vi "Pre Launch Init.vi"(11 "UI in":refnum<class "UI.lvclass">) -> (0 "error out":errorcluster, 3 "UI out":refnum<class "UI.lvclass">)   [LabVIEW 2020, in "UI.lvlib" / "UI.lvclass"]
doc: "<p>(<strong>Filename</strong>: <span class=\"dnl\">Actor Framework.lvlib:Actor.lvclass:Pre Launch Init.vi</span>)</p>\n<p>Defines behavior that occurs after the <a href=\"nihelplauncher://docs/csh?context=lvcore_lvcomm_af_launch_nested_actor\">Launch Nested Actor</a> method is invoked but before the actor's Actor Core method begins running.</p>\n<p>By default, this method does nothing. A descendant class may override it to define behavior.</p>"
uses:
  UI.lvclass
  UI.lvclass/UI.ctl
  <vilib>/ActorFramework/Actor/Actor.lvclass
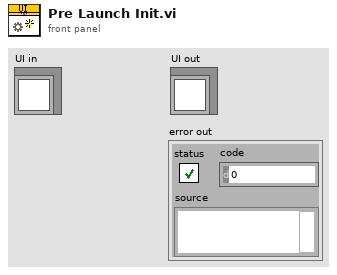
[diagram p1: front panel]
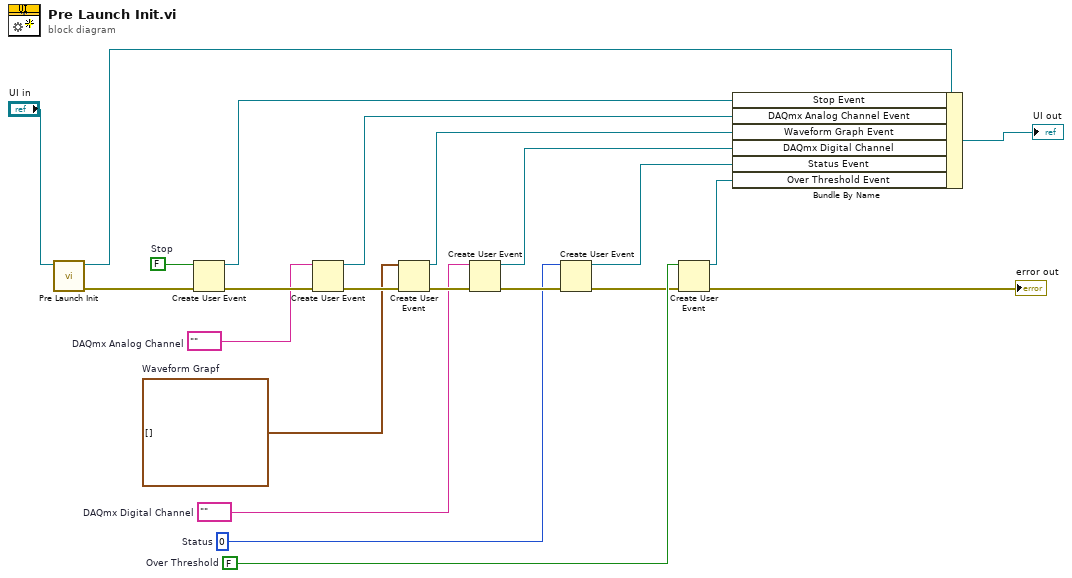
[diagram p0: block diagram]
diagram:
  w4 = FALSE  # Over Threshold
  w6 = waveform(dbl)[] []  # Waveform Grapf
  w8 = u8 0  # Status
  w10 = tag ""  # DAQmx Digital Channel
  w12 = tag ""  # DAQmx Analog Channel
  w14 = FALSE  # Stop
  n1 = call-parent "Pre Launch Init.vi"("Actor in"="UI in") -> ("error out"=w15:errorcluster, "Actor out"=w21:refnum<class "UI.lvclass">)  [unwired: 9 in]
  n2 = Create User Event(user event datatype=w14, error in=w15) -> (user event=w13:refnum<user-event>, error out=w19:errorcluster)
  n3 = Create User Event(user event datatype=w12, error in=w19) -> (user event=w11:refnum<user-event>, error out=w18:errorcluster)
  n4 = Create User Event(user event datatype=w6, error in=w18) -> (user event=w5:refnum<user-event>, error out=w17:errorcluster)
  n5 = Create User Event(user event datatype=w10, error in=w17) -> (user event=w9:refnum<user-event>, error out=w16:errorcluster)
  n6 = Create User Event(user event datatype=w8, error in=w16) -> (user event=w7:refnum<user-event>, error out=w3:errorcluster)
  n7 = Create User Event(user event datatype=w4, error in=w3) -> (user event=w2:refnum<user-event>, error out=→"error out":errorcluster)
  n8 = Bundle By Name(cluster=w21, "Stop Event"=w13, "DAQmx Analog Channel Event"=w11, "Waveform Graph Event"=w5, "DAQmx Digital Channel"=w9, "Status Event"=w7, "Over Threshold Event"=w2) -> (→"UI out":refnum<class "UI.lvclass">)
